vi "Caller.vi"(6 "Sub Panel":refnum<vi>, 8 "Error In":errorcluster, 10 "Data Value Reference In":refnum<data-value>, 11 "Subtract In":refnum<class "Subtract.lvclass">) -> (0 "Error Out":errorcluster, 3 "Subtract Out":refnum<class "Subtract.lvclass">)   [LabVIEW 2021, in "Calculator.lvlib" / "Subtract.lvclass"]
doc: "This VI is an overriding method which asynchronously calls the UI.vi"
uses:
  Subtract.lvclass
  UI.vi
  NumericOperation/NumericOperation.lvclass
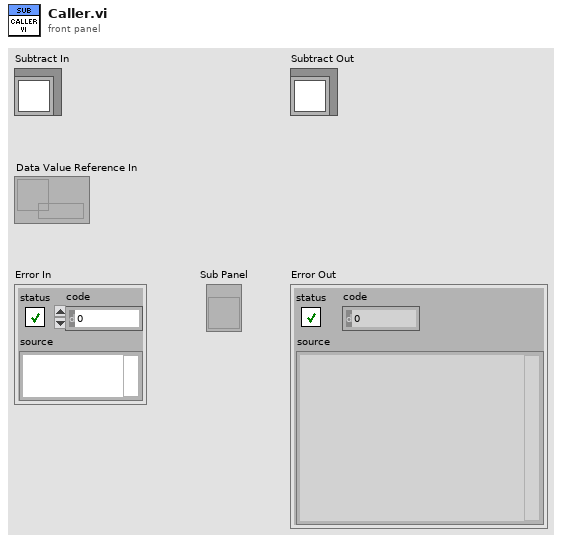
[diagram p1: front panel]
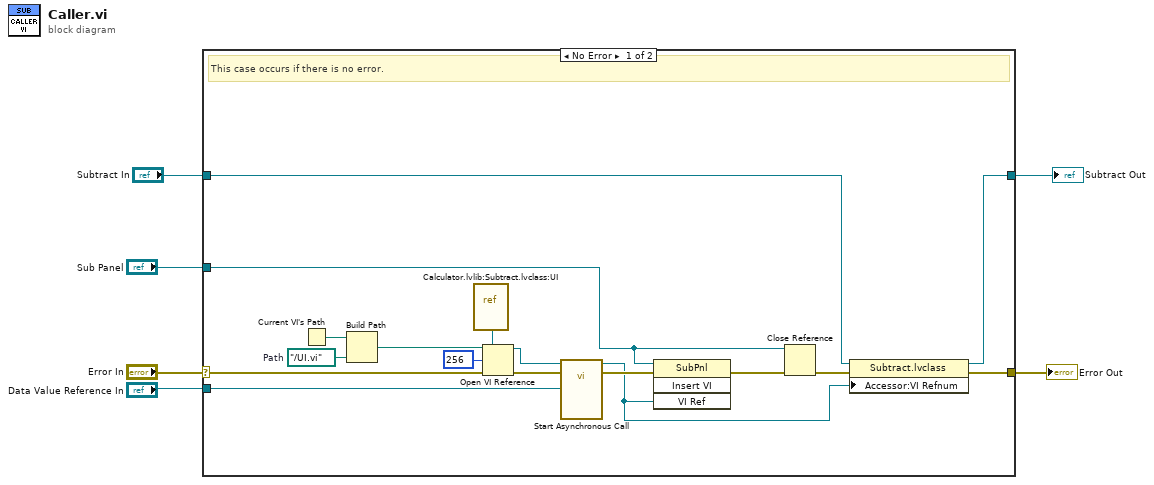
[diagram p0: block diagram]
diagram:
  n1 = case shown="No Error" "Error In" {
    selector: "Error In" -> [w23 w25]
    tunnel: [w14 w25] -> w5
    tunnel: [w12 w24] -> w3
    tunnel: "Subtract In" -> [w13 w24]
    tunnel: "Sub Panel" -> [w9 _]
    tunnel: "Data Value Reference In" -> [w7 _]
    frame No Error {
      w19 = path "../UI.vi"  # Path
      # "This case occurs if there is no error."
      n2 = Current VI's Path() -> (path=w20:path)
      n3 = Build Path(base path=w20, name or relative path=w19) -> (appended path=w18:path)
      n4 = vi-ref "Calculator.lvlib:Subtract.lvclass:UI.vi"() -> (w17:refnum<vi>)
      n5 = Open VI Reference(type specifier VI Refnum (for type only)=w17, vi path=w18, options=256, error in (no error)=w23) -> (vi reference=w16:refnum<vi>, error out=w22:errorcluster)  [unwired: 2 in]
      n6 = call-by-ref "Start Asynchronous Call"(reference=w16, error in=w22, "Data Value Reference In"=w7) -> (reference out=w8:refnum<vi>, error out=w21:errorcluster)  [unwired: 8 in, 3 out]
      n7 = invoke class="SubPnl" method="Insert VI"(reference=w9, error in=w21, "VI Ref"=w8) -> (error out=w10:errorcluster)  [unwired: 1 in, 3 out]
      n8 = Close Reference(reference=w9, error in (no error)=w10) -> (error out=w11:errorcluster)
      n9 = property class="Subtract.lvclass"(reference=w13, error in=w11, "Accessor:VI Refnum"=w8) -> (reference out=w12:refnum<class "Subtract.lvclass">, error out=w14:errorcluster)
    }
    frame Error {
      # "This case occurs if there is any error."
    }
  }
  "Error Out" <- w5
  "Subtract Out" <- w3
